vi "Stream Data I16x1.vi"(0 "i in":fxp<+/-,18,1>, 7 "config":T3, 9 "input valid":bool) -> (6 "status":T2)   [LabVIEW 2017, in "Lock-In Amplifier Example FPGA.lvlib"]
uses:
  Lock-In Amplifier Example FPGA.lvlib
  <instrlib>/_niInstr/Streaming/v1/Common/Stream State.ctl
  <vilib>/rvi/interface/RandomDataEmulation/niFpgaRandomDataHandleErrors.vi
  <vilib>/rvi/DataTransferAndStorage/Container/XNode/niFpgaContainer.xnode
  <vilib>/rvi/interface/RandomDataEmulation/nirviRandomDataFpgaReadWriteTemplate.vi
  <instrlib>/_niInstr/Streaming/v1/FPGA/niInstr Streaming v1 FPGA.lvlib
  <instrlib>/_niInstr/Streaming/v1/Common/niInstr Streaming v1 Common.lvlib
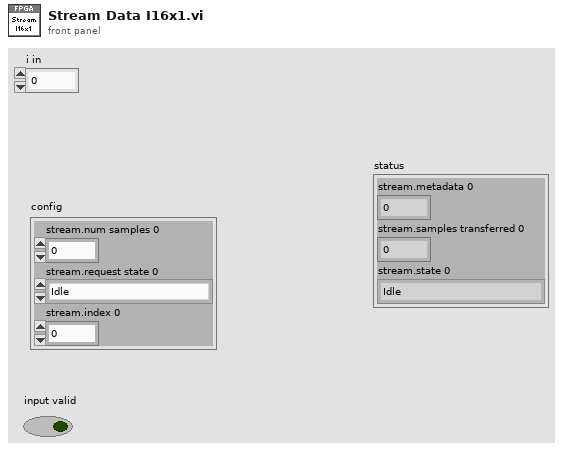
[diagram p1: front panel]
types:
  T1 = typedef "niInstr Streaming v1 Common.lvlib/Stream State.ctl" = enum8{"Idle", "Finite Transfer", "Continuous", "Done", "Error", "Not Ready", "Cancel"}
  T2 = cluster{"stream.metadata 0":u64, "stream.samples transferred 0":u64, "stream.state 0":T1}
  T3 = cluster{"stream.num samples 0":u64, "stream.request state 0":T1, "stream.index 0":i16}
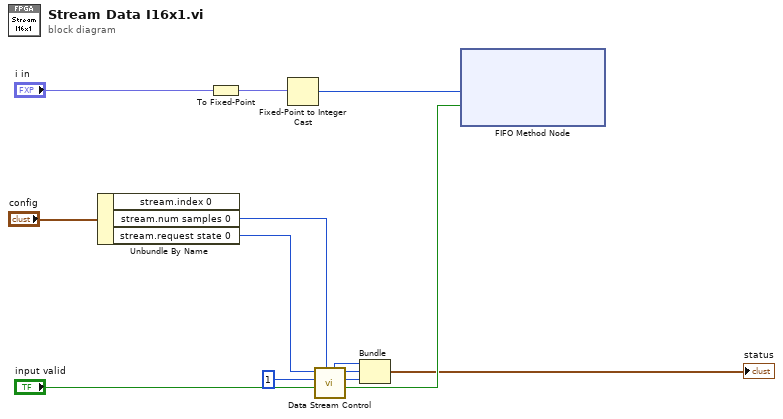
[diagram p0: block diagram]
diagram:
  n1 = Unbundle By Name("config") -> ("stream.num samples 0"=w7:u64, "stream.request state 0"=w6:T1)  [unwired: 1 out]
  n2 = To Fixed-Point(number="i in") -> (fixed-point=w1:fxp<+/-,16,1>)  [unwired: 1 in]
  n3 = Fixed-Point to Integer Cast(1:w1) -> (0:w10:i16)
  n4 = call <instrlib>:"Data Stream Control.vi"("stream.num samples 0"=w7, "data valid"="input valid", "element count"=u16 1, "stream.request state 0"=w6) -> ("send data"=w9:bool, "stream.state 0"=w3:T1, "stream.samples transferred 0"=w4:u64, "stream.metadata 0"=w5:u64)  [unwired: 3 in, 1 out]
  n5 = Bundle("stream.metadata 0"=w5, "stream.samples transferred 0"=w4, "stream.state 0"=w3) -> (→"status":T2)  [unwired: 1 in]
  n6 = xnode ("FIFO Method Node")("Element"=w10, "Input Valid"=w9) -> ()  [unwired: 1 in, 2 out]
